vi "Prueba GAP.vi"(11 "Class 2.lvclass":refnum<class "Class 2.lvclass">) -> (3 "Class 2.lvclass 2":refnum<class "Class 2.lvclass">)   [LabVIEW 2019, in "Class 2.lvclass"]
uses:
  Class 2.lvclass
  Class 2.lvclass/Class 2.ctl
panel:
  in  "stop":bool
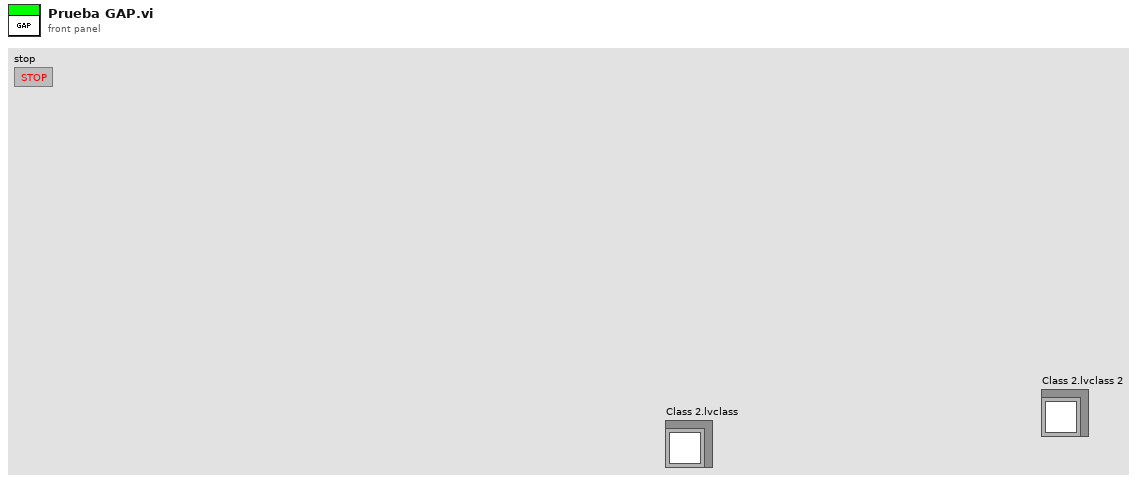
[diagram p1: front panel]
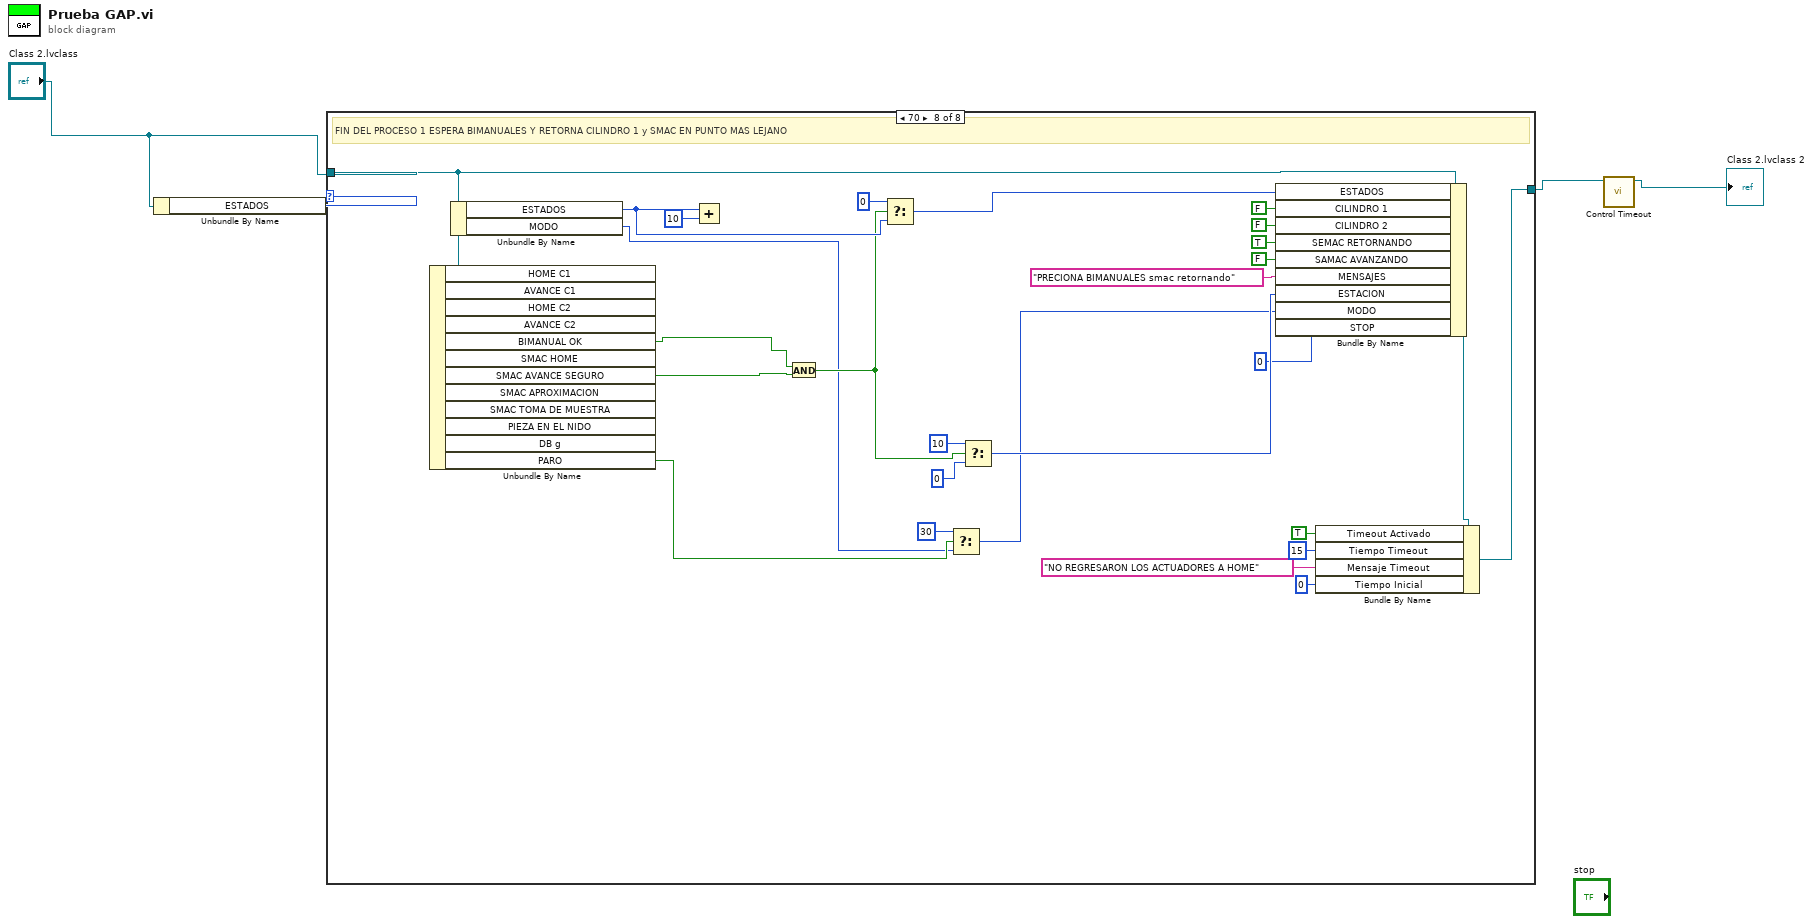
[diagram p0: block diagram]
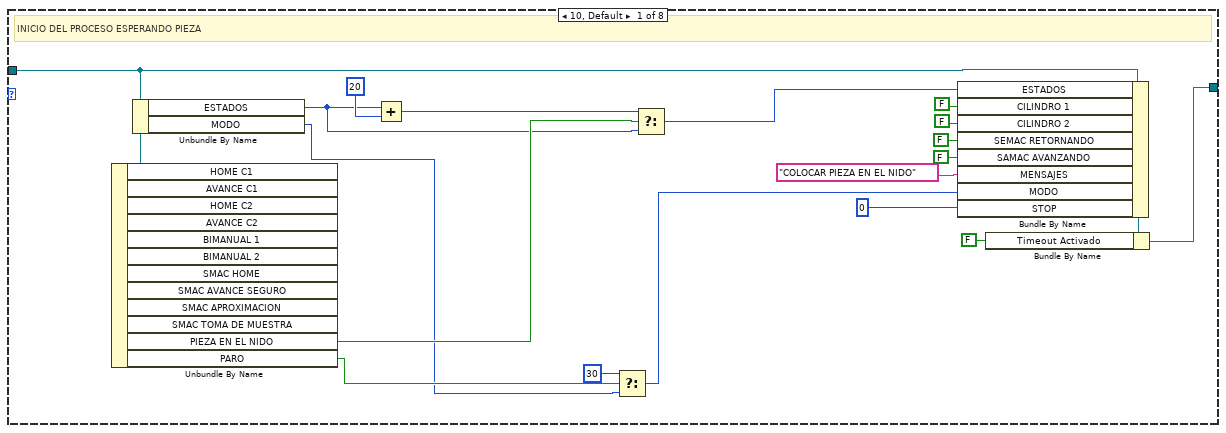
[diagram p2: hidden frame]
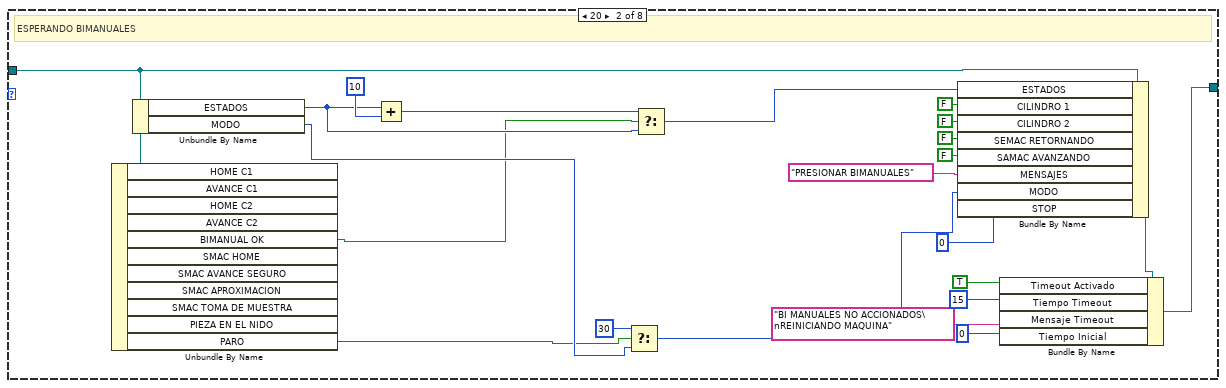
[diagram p3: hidden frame]
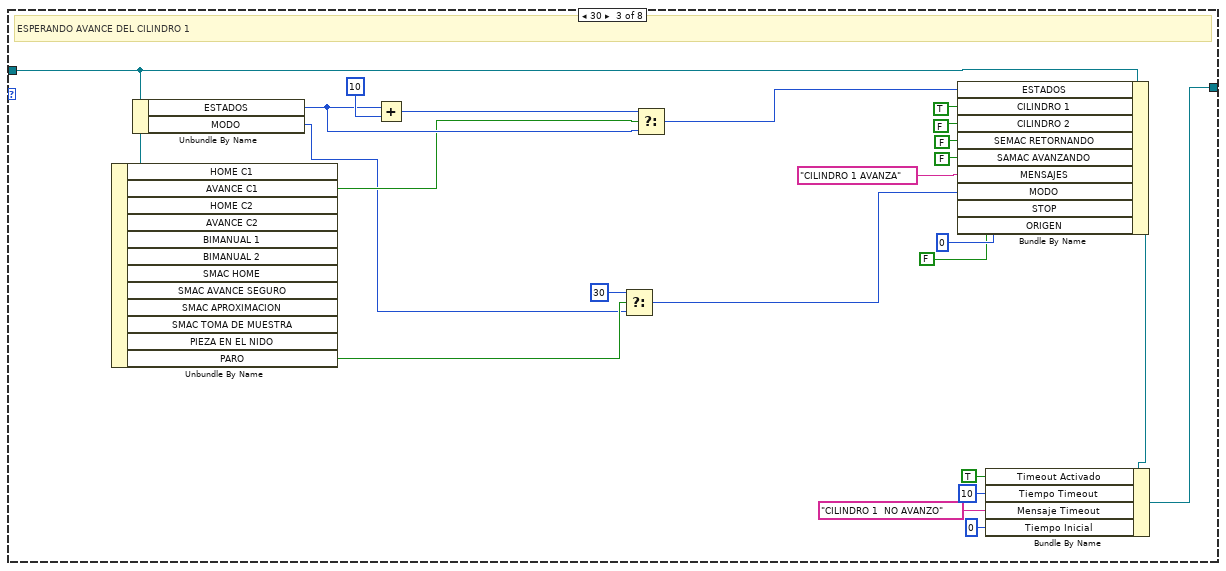
[diagram p4: hidden frame]
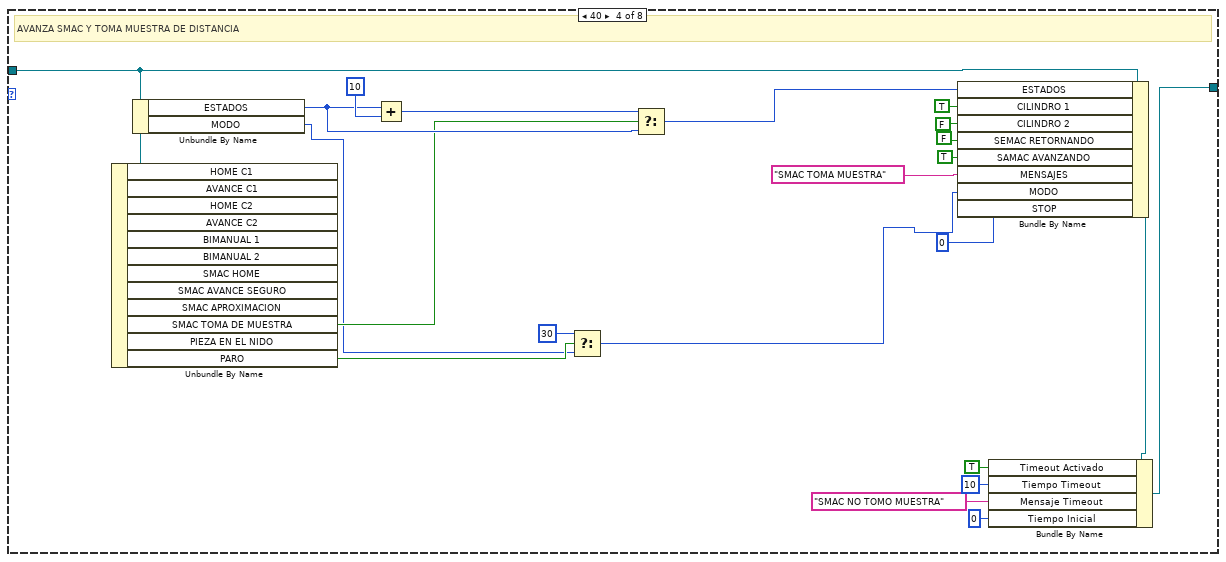
[diagram p5: hidden frame]
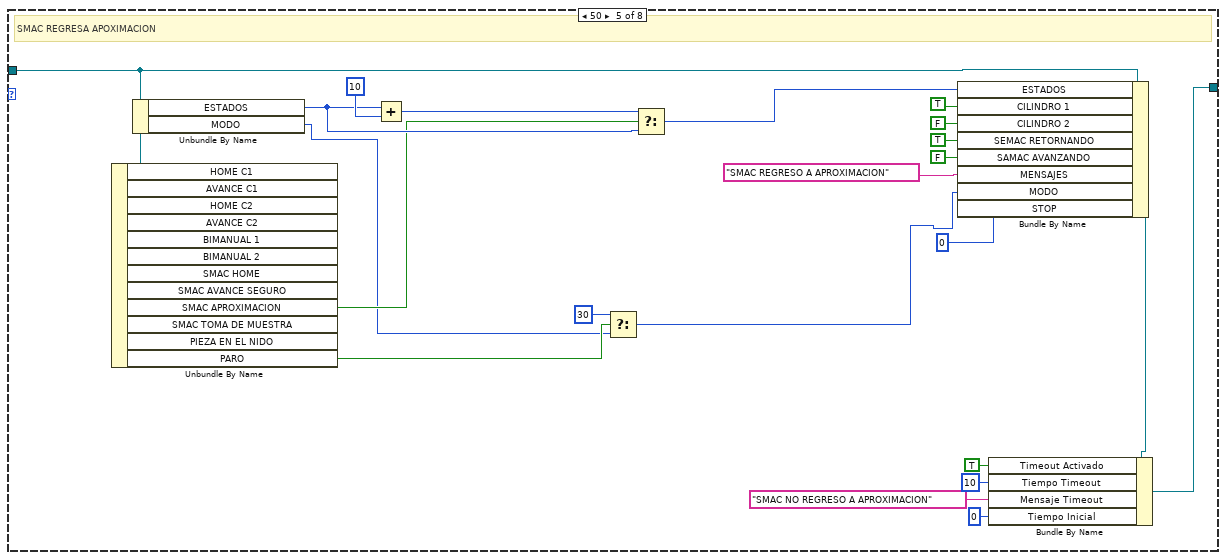
[diagram p6: hidden frame]
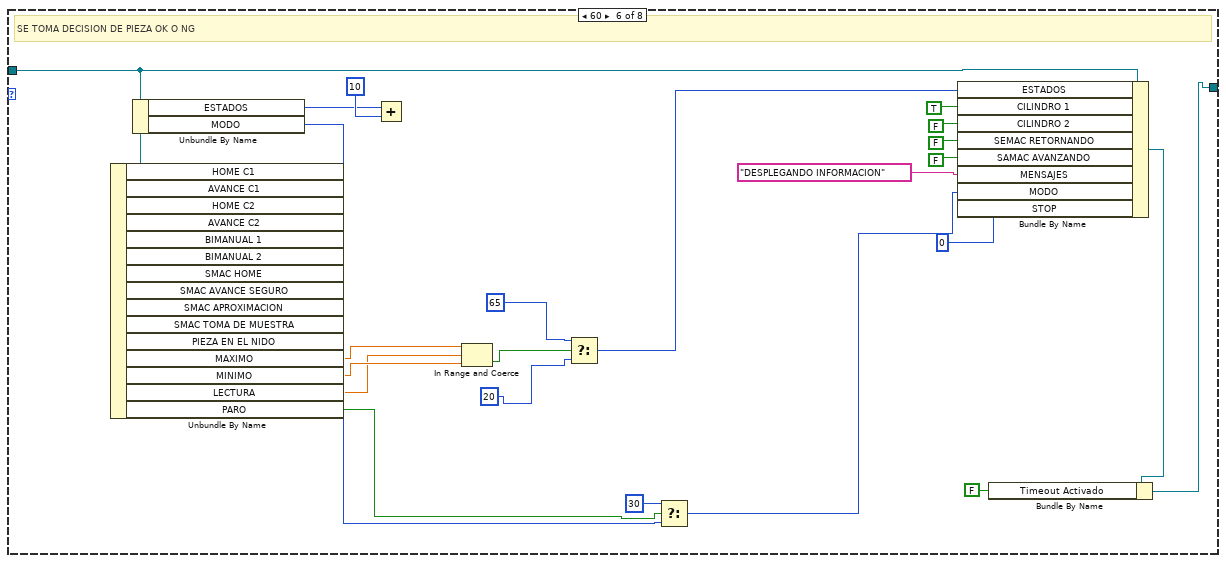
[diagram p7: hidden frame]
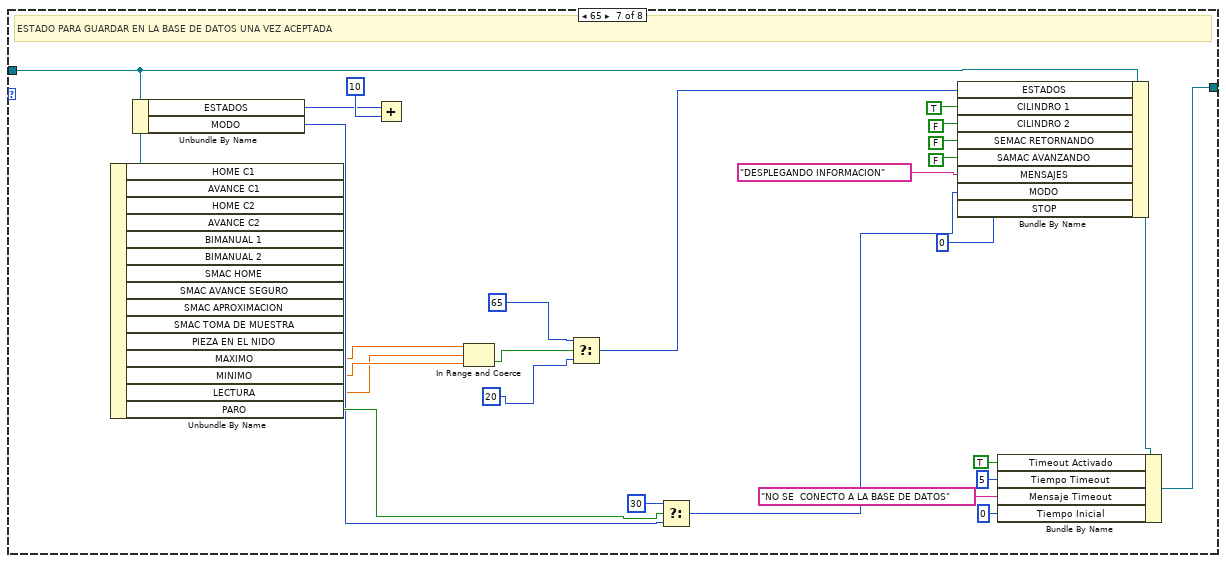
[diagram p8: hidden frame]
diagram:
  n1 = Unbundle By Name("Class 2.lvclass") -> ("ESTADOS"=w4:i16)
  n2 = case shown="70" w4 {
    tunnel: "Class 2.lvclass" -> [w20 w41 w64 w86 w108 w134 w160 w187]
    tunnel: [w6 w24 w46 w69 w91 w113 w136 w162] -> w2
    frame 10, Default {
      # "INICIO DEL PROCESO ESPERANDO PIEZA"
      n3 = Unbundle By Name(w20) -> ("PIEZA EN EL NIDO"=w18:bool, "PARO"=w13:bool)  [unwired: 10 out]
      n4 = Unbundle By Name(w20) -> ("ESTADOS"=w12:i16, "MODO"=w10:i16)
      n5 = Add(x=w12, y=i16 20) -> (x+y=w22:i16)
      n6 = Select(t=i16 30, s=w13, f=w10) -> (s? t:f=w8:i16)
      n7 = Select(t=w22, s=w18, f=w12) -> (s? t:f=w21:i16)
      n8 = Bundle By Name(cluster=w20, "ESTADOS"=w21, "CILINDRO 1"=FALSE ("SALIDAS.CILINDRO 1"), "CILINDRO 2"=FALSE ("SALIDAS.CILINDRO 2"), "SEMAC RETORNANDO"=FALSE ("SALIDAS.SEMAC RETORNANDO"), "SAMAC AVANZANDO"=FALSE ("SALIDAS.SAMAC AVANZANDO"), "MENSAJES"="COLOCAR PIEZA EN EL NIDO" ("SALIDAS.MENSAJES"), "MODO"=w8, "STOP"=i16 0 ("MAQ DE ESTADOS.MODO")) -> (w7:refnum<class "Class 2.lvclass">)
      n9 = Bundle By Name(cluster=w7, "Timeout Activado"=FALSE ("Timeout.Timeout Activado")) -> (w6:refnum<class "Class 2.lvclass">)
    }
    frame 20 {
      # "ESPERANDO BIMANUALES"
      n10 = Unbundle By Name(w41) -> ("BIMANUAL OK"=w30:bool, "PARO"=w33:bool)  [unwired: 9 out]
      n11 = Unbundle By Name(w41) -> ("ESTADOS"=w43:i16, "MODO"=w34:i16)
      n12 = Add(x=w43, y=i16 10) -> (x+y=w44:i16)
      n13 = Select(t=i16 30, s=w33, f=w34) -> (s? t:f=w32:i16)
      n14 = Select(t=w44, s=w30, f=w43) -> (s? t:f=w42:i16)
      n15 = Bundle By Name(cluster=w41, "ESTADOS"=w42, "CILINDRO 1"=FALSE ("SALIDAS.CILINDRO 1"), "CILINDRO 2"=FALSE ("SALIDAS.CILINDRO 2"), "SEMAC RETORNANDO"=FALSE ("SALIDAS.SEMAC RETORNANDO"), "SAMAC AVANZANDO"=FALSE ("SALIDAS.SAMAC AVANZANDO"), "MENSAJES"="PRESIONAR BIMANUALES" ("SALIDAS.MENSAJES"), "MODO"=w32, "STOP"=i16 0 ("MAQ DE ESTADOS.STOP")) -> (w25:refnum<class "Class 2.lvclass">)
      n16 = Bundle By Name(cluster=w25, "Timeout Activado"=TRUE ("Timeout.Timeout Activado"), "Tiempo Timeout"=u32 15 ("Timeout.Tiempo Timeout"), "Mensaje Timeout"="BI MANUALES NO ACCIONADOS\nREINICIANDO MAQUINA" ("Timeout.Mensaje Timeout"), "Tiempo Inicial"=u32 0 ("Timeout.Tiempo Inicial")) -> (w24:refnum<class "Class 2.lvclass">)
    }
    frame 30 {
      # "ESPERANDO AVANCE DEL CILINDRO 1"
      n17 = Unbundle By Name(w64) -> ("AVANCE C1"=w58:bool, "PARO"=w55:bool)  [unwired: 10 out]
      n18 = Unbundle By Name(w64) -> ("ESTADOS"=w66:i16, "MODO"=w54:i16)
      n19 = Add(x=w66, y=i16 10) -> (x+y=w67:i16)
      n20 = Select(t=i16 30, s=w55, f=w54) -> (s? t:f=w56:i16)
      n21 = Select(t=w67, s=w58, f=w66) -> (s? t:f=w65:i16)
      n22 = Bundle By Name(cluster=w64, "ESTADOS"=w65, "CILINDRO 1"=TRUE ("SALIDAS.CILINDRO 1"), "CILINDRO 2"=FALSE ("SALIDAS.CILINDRO 2"), "SEMAC RETORNANDO"=FALSE ("SALIDAS.SEMAC RETORNANDO"), "SAMAC AVANZANDO"=FALSE ("SALIDAS.SAMAC AVANZANDO"), "MENSAJES"="CILINDRO 1 AVANZA" ("SALIDAS.MENSAJES"), "MODO"=w56, "STOP"=i16 0 ("MAQ DE ESTADOS.STOP"), "ORIGEN"=FALSE ("PROCESO.ORIGEN")) -> (w47:refnum<class "Class 2.lvclass">)
      n23 = Bundle By Name(cluster=w47, "Timeout Activado"=TRUE ("Timeout.Timeout Activado"), "Tiempo Timeout"=u32 10 ("Timeout.Tiempo Timeout"), "Mensaje Timeout"="CILINDRO 1  NO AVANZO" ("Timeout.Mensaje Timeout"), "Tiempo Inicial"=u32 0 ("Timeout.Tiempo Inicial")) -> (w46:refnum<class "Class 2.lvclass">)
    }
    frame 40 {
      # "AVANZA SMAC Y TOMA MUESTRA DE DISTANCIA"
      n24 = Unbundle By Name(w86) -> ("SMAC TOMA DE MUESTRA"=w80:bool, "PARO"=w78:bool)  [unwired: 10 out]
      n25 = Unbundle By Name(w86) -> ("ESTADOS"=w88:i16, "MODO"=w77:i16)
      n26 = Add(x=w88, y=i16 10) -> (x+y=w89:i16)
      n27 = Select(t=i16 30, s=w78, f=w77) -> (s? t:f=w76:i16)
      n28 = Select(t=w89, s=w80, f=w88) -> (s? t:f=w87:i16)
      n29 = Bundle By Name(cluster=w86, "ESTADOS"=w87, "CILINDRO 1"=TRUE ("SALIDAS.CILINDRO 1"), "CILINDRO 2"=FALSE ("SALIDAS.CILINDRO 2"), "SEMAC RETORNANDO"=FALSE ("SALIDAS.SEMAC RETORNANDO"), "SAMAC AVANZANDO"=TRUE ("SALIDAS.SAMAC AVANZANDO"), "MENSAJES"="SMAC TOMA MUESTRA" ("SALIDAS.MENSAJES"), "MODO"=w76, "STOP"=i16 0 ("MAQ DE ESTADOS.STOP")) -> (w70:refnum<class "Class 2.lvclass">)
      n30 = Bundle By Name(cluster=w70, "Timeout Activado"=TRUE ("Timeout.Timeout Activado"), "Tiempo Timeout"=u32 10 ("Timeout.Tiempo Timeout"), "Mensaje Timeout"="SMAC NO TOMO MUESTRA" ("Timeout.Mensaje Timeout"), "Tiempo Inicial"=u32 0 ("Timeout.Tiempo Inicial")) -> (w69:refnum<class "Class 2.lvclass">)
    }
    frame 50 {
      # "SMAC REGRESA APOXIMACION"
      n31 = Unbundle By Name(w108) -> ("SMAC APROXIMACION"=w102:bool, "PARO"=w100:bool)  [unwired: 10 out]
      n32 = Unbundle By Name(w108) -> ("ESTADOS"=w110:i16, "MODO"=w99:i16)
      n33 = Add(x=w110, y=i16 10) -> (x+y=w111:i16)
      n34 = Select(t=i16 30, s=w100, f=w99) -> (s? t:f=w98:i16)
      n35 = Select(t=w111, s=w102, f=w110) -> (s? t:f=w109:i16)
      n36 = Bundle By Name(cluster=w108, "ESTADOS"=w109, "CILINDRO 1"=TRUE ("SALIDAS.CILINDRO 1"), "CILINDRO 2"=FALSE ("SALIDAS.CILINDRO 2"), "SEMAC RETORNANDO"=TRUE ("SALIDAS.SEMAC RETORNANDO"), "SAMAC AVANZANDO"=FALSE ("SALIDAS.SAMAC AVANZANDO"), "MENSAJES"="SMAC REGRESO A APROXIMACION" ("SALIDAS.MENSAJES"), "MODO"=w98, "STOP"=i16 0 ("MAQ DE ESTADOS.STOP")) -> (w92:refnum<class "Class 2.lvclass">)
      n37 = Bundle By Name(cluster=w92, "Timeout Activado"=TRUE ("Timeout.Timeout Activado"), "Tiempo Timeout"=u32 10 ("Timeout.Tiempo Timeout"), "Mensaje Timeout"="SMAC NO REGRESO A APROXIMACION" ("Timeout.Mensaje Timeout"), "Tiempo Inicial"=u32 0 ("Timeout.Tiempo Inicial")) -> (w91:refnum<class "Class 2.lvclass">)
    }
    frame 60 {
      # "SE TOMA DECISION DE PIEZA OK O NG"
      n38 = Unbundle By Name(w134) -> ("MAXIMO"=w122:dbl, "MINIMO"=w121:dbl, "LECTURA"=w120:dbl, "PARO"=w126:bool)  [unwired: 11 out]
      n39 = Unbundle By Name(w134) -> ("ESTADOS"=w128:i16, "MODO"=w125:i16)
      n40 = Add(x=w128, y=i16 10) -> ()  [unwired: 1 out]
      n41 = In Range and Coerce(upper limit=w122, x=w120, lower limit=w121) -> (In Range?=w119:bool)  [unwired: 1 out]
      n42 = Select(t=i16 65 ("y"), s=w119, f=i16 20 ("y")) -> (s? t:f=w116:i16)
      n43 = Select(t=i16 30, s=w126, f=w125) -> (s? t:f=w124:i16)
      n44 = Bundle By Name(cluster=w134, "ESTADOS"=w116, "CILINDRO 1"=TRUE ("SALIDAS.CILINDRO 1"), "CILINDRO 2"=FALSE ("SALIDAS.CILINDRO 2"), "SEMAC RETORNANDO"=FALSE ("SALIDAS.SEMAC RETORNANDO"), "SAMAC AVANZANDO"=FALSE ("SALIDAS.SAMAC AVANZANDO"), "MENSAJES"="DESPLEGANDO INFORMACION" ("SALIDAS.MENSAJES"), "MODO"=w124, "STOP"=i16 0 ("MAQ DE ESTADOS.STOP")) -> (w114:refnum<class "Class 2.lvclass">)
      n45 = Bundle By Name(cluster=w114, "Timeout Activado"=FALSE ("Timeout.Timeout Activado")) -> (w113:refnum<class "Class 2.lvclass">)
    }
    frame 65 {
      # "ESTADO PARA GUARDAR EN LA BASE DE DATOS UNA VEZ ACEPTADA"
      n46 = Unbundle By Name(w160) -> ("MAXIMO"=w148:dbl, "MINIMO"=w147:dbl, "LECTURA"=w146:dbl, "PARO"=w152:bool)  [unwired: 11 out]
      n47 = Unbundle By Name(w160) -> ("ESTADOS"=w154:i16, "MODO"=w151:i16)
      n48 = Add(x=w154, y=i16 10) -> ()  [unwired: 1 out]
      n49 = In Range and Coerce(upper limit=w148, x=w146, lower limit=w147) -> (In Range?=w145:bool)  [unwired: 1 out]
      n50 = Select(t=i16 65 ("y"), s=w145, f=i16 20 ("y")) -> (s? t:f=w142:i16)
      n51 = Select(t=i16 30, s=w152, f=w151) -> (s? t:f=w150:i16)
      n52 = Bundle By Name(cluster=w160, "ESTADOS"=w142, "CILINDRO 1"=TRUE ("SALIDAS.CILINDRO 1"), "CILINDRO 2"=FALSE ("SALIDAS.CILINDRO 2"), "SEMAC RETORNANDO"=FALSE ("SALIDAS.SEMAC RETORNANDO"), "SAMAC AVANZANDO"=FALSE ("SALIDAS.SAMAC AVANZANDO"), "MENSAJES"="DESPLEGANDO INFORMACION" ("SALIDAS.MENSAJES"), "MODO"=w150, "STOP"=i16 0 ("MAQ DE ESTADOS.STOP")) -> (w137:refnum<class "Class 2.lvclass">)
      n53 = Bundle By Name(cluster=w137, "Timeout Activado"=TRUE ("Timeout.Timeout Activado"), "Tiempo Timeout"=u32 5 ("Timeout.Tiempo Timeout"), "Mensaje Timeout"="NO SE  CONECTO A LA BASE DE DATOS" ("Timeout.Mensaje Timeout"), "Tiempo Inicial"=u32 0 ("Timeout.Tiempo Inicial")) -> (w136:refnum<class "Class 2.lvclass">)
    }
    frame 70 {
      # "FIN DEL PROCESO 1 ESPERA BIMANUALES Y RETORNA CILINDRO 1 y SMAC EN PUNTO MAS LEJANO"
      n54 = Unbundle By Name(w187) -> ("BIMANUAL OK"=w168:bool, "SMAC AVANCE SEGURO"=w178:bool, "PARO"=w172:bool)  [unwired: 9 out]
      n55 = Unbundle By Name(w187) -> ("ESTADOS"=w180:i16, "MODO"=w171:i16)
      n56 = Add(x=w180, y=i16 10) -> ()  [unwired: 1 out]
      n57 = And(x=w168, y=w178) -> (x .and. y?=w176:bool)
      n58 = Select(t=i16 0, s=w176, f=w180) -> (s? t:f=w181:i16)
      n59 = Select(t=i16 30, s=w172, f=w171) -> (s? t:f=w169:i16)
      n60 = Select(t=i8 10, s=w176, f=i8 0) -> (s? t:f=w174:i8)
      n61 = Bundle By Name(cluster=w187, "ESTADOS"=w181, "CILINDRO 1"=FALSE ("SALIDAS.CILINDRO 1"), "CILINDRO 2"=FALSE ("SALIDAS.CILINDRO 2"), "SEMAC RETORNANDO"=TRUE ("SALIDAS.SEMAC RETORNANDO"), "SAMAC AVANZANDO"=FALSE ("SALIDAS.SAMAC AVANZANDO"), "MENSAJES"="PRECIONA BIMANUALES smac retornando" ("SALIDAS.MENSAJES"), "ESTACION"=w174, "MODO"=w169, "STOP"=i16 0 ("MAQ DE ESTADOS.STOP")) -> (w163:refnum<class "Class 2.lvclass">)
      n62 = Bundle By Name(cluster=w163, "Timeout Activado"=TRUE ("Timeout.Timeout Activado"), "Tiempo Timeout"=u32 15 ("Timeout.Tiempo Timeout"), "Mensaje Timeout"="NO REGRESARON LOS ACTUADORES A HOME" ("Timeout.Mensaje Timeout"), "Tiempo Inicial"=u32 0 ("Timeout.Tiempo Inicial")) -> (w162:refnum<class "Class 2.lvclass">)
    }
  }
  n63 = call "Control Timeout.vi"("Class 2 in"=w2) -> ("Class 2 out"=→"Class 2.lvclass 2":refnum<class "Class 2.lvclass">)  [unwired: 10 in]
